vi "Decimation FG.vi"(7 "Action":T1, 8 "error in (no error)":errorcluster, 10 "Decimation":u32=1, 11 "Device Item Ref in":T2 format="%.0x") -> (0 "error out":errorcluster, 2 "Decimation out":u32, 3 "Item Ref out":T2 format="%.0x")   [LabVIEW 2019, in "Instrument Addon Shared.lvlib"]
uses:
  Instrument Addon Shared.lvlib
  <vilib>/NI VeriStand/Custom Device API/Custom Device Item Ref.ctl
  Types/FG Control.ctl
  Constants.vi
  <vilib>/NI VeriStand/Custom Device API/Get Item Property (U32).vi
  <vilib>/NI VeriStand/Custom Device API/Set Item Property (U32).vi
  <vilib>/NI VeriStand/Custom Device API/Custom Device API.lvlib
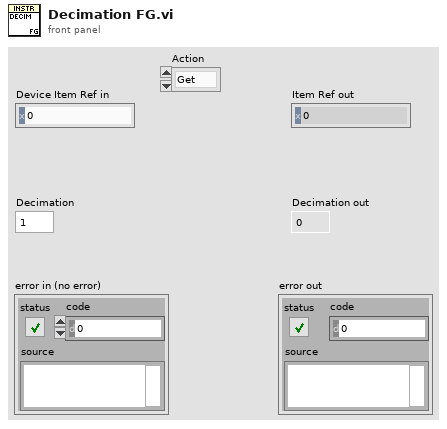
[diagram p1: front panel]
types:
  T1 = typedef "Instrument Addon Shared.lvlib/FG Control.ctl" = enum16{"Get", "Set"}
  T2 = typedef "Custom Device API.lvlib/Custom Device Item Ref.ctl" = u64
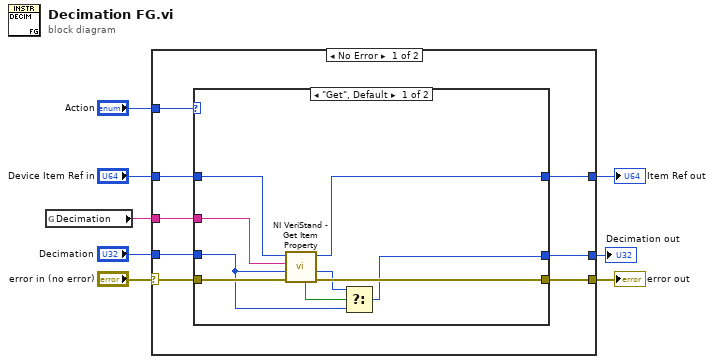
[diagram p0: block diagram]
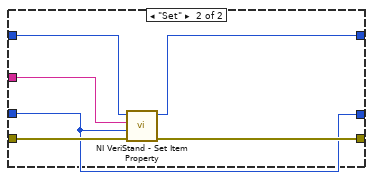
[diagram p2: hidden frame]
diagram:
  n1 = global read "Constants.vi" "Decimation"() -> (w8:string)
  n2 = case shown="No Error" "error in (no error)" {
    selector: "error in (no error)" -> [w11 w34]
    tunnel: w8 -> [w16 _]
    tunnel: [w15 w32] -> w7
    tunnel: "Device Item Ref in" -> [w14 w32]
    tunnel: "Decimation" -> [w13 w33]
    tunnel: [w12 w34] -> w4
    tunnel: [w10 w33] -> w2
    tunnel: "Action" -> [w9 _]
    frame No Error {
      n3 = case shown="\"Get\", Default" w9 {
        tunnel: w16 -> [w22 w31]
        tunnel: [w23 w30] -> w15
        tunnel: w14 -> [w24 w29]
        tunnel: w13 -> [w19 w26]
        tunnel: [w21 w28] -> w12
        tunnel: w11 -> [w25 w27]
        tunnel: [w17 w26] -> w10
        frame "Get", Default {
          n4 = call-poly <vilib>:"NI VeriStand - Get Item Property.vi"("error in (no error)"=w25, "Default Value"=w19, "Property Name"=w22, "Item Ref in"=w24) -> ("error out"=w21:errorcluster, "Value"=w18:u32, "Item Ref out"=w23:T2, "Found?"=w20:bool)  [unwired: 4 in]
          n5 = Select(t=w18, s=w20, f=w19) -> (s? t:f=w17:u32)
        }
        frame "Set" {
          n6 = call-poly <vilib>:"NI VeriStand - Set Item Property.vi"("error in (no error)"=w27, "Value"=w26, "Property Name"=w31, "Item Ref in"=w29) -> ("error out"=w28:errorcluster, "Item Ref out"=w30:T2)  [unwired: 5 in, 1 out]
        }
      }
    }
    frame Error {
    }
  }
  "Item Ref out" <- w7
  "error out" <- w4
  "Decimation out" <- w2
